vi "Get Slaves.vi"(8 "error in (no error)":errorcluster, 11 "EtherCAT Master in":T3 {"VS ref" format="%.0x"}) -> (0 "error out":errorcluster, 1 "ECAT Generic Slaves":T2(array[cluster]) {"VS ref" format="%.0x"}, 2 "ECAT Slaves":T2(array[cluster]) {"VS ref" format="%.0x"}, 3 "EtherCAT Master out":T3 {"VS ref" format="%.0x"}, 4 "ECAT REM Slaves":T2(array[cluster]) {"VS ref" format="%.0x"})   [LabVIEW 2019, in "SEECD Engine.lvlib"]
uses:
  SEECD Engine.lvlib
  <vilib>/NI VeriStand/Custom Device API/Custom Device Item Ref.ctl
  Shared/Globals/Scan Engine GUIDs.vi
  <vilib>/NI VeriStand/Custom Device API/Custom Device API.lvlib
  Shared/SEECD Shared.lvlib
  <resource>/objmgr/IndComECAT.rc
  <vilib>/NI VeriStand/Custom Device Tools/Custom Device Utility Library/Custom Device Utility Library.lvlib
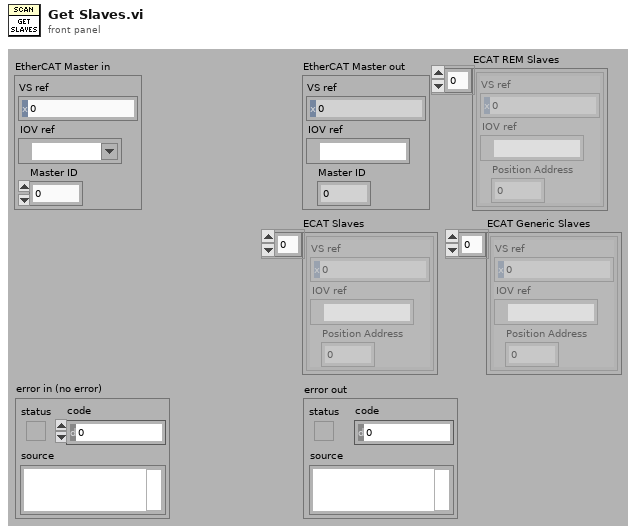
[diagram p1: front panel]
types:
  T1 = typedef "Custom Device API.lvlib/Custom Device Item Ref.ctl" = u64
  T2 = cluster{"VS ref":T1, "IOV ref":refnum<k21>, "Position Address":u16}[]
  T3 = cluster{"VS ref":T1, "IOV ref":refnum<k21>, "Master ID":u32}
  T4 = cluster{"ECAT Slave refs":T1[], "All ECAT Slaves":refnum<k21>[]}
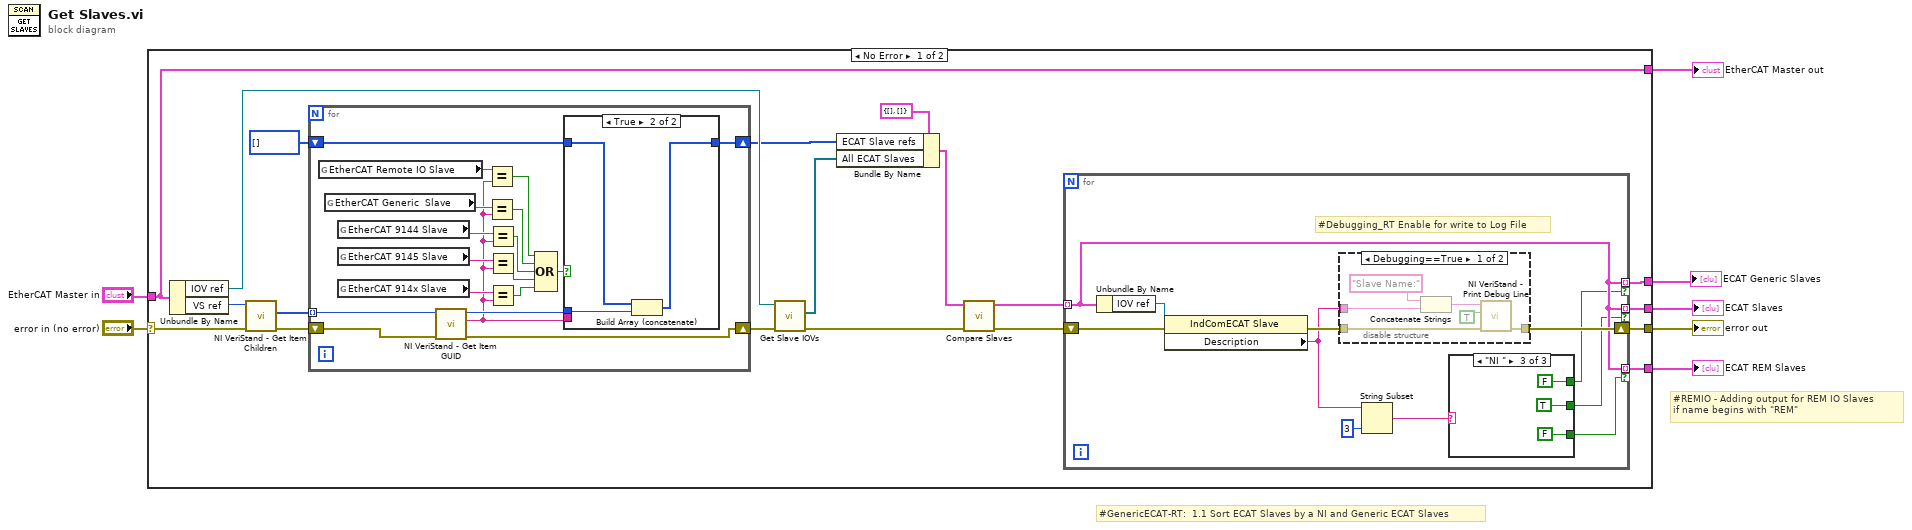
[diagram p0: block diagram]
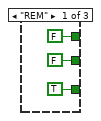
[diagram p3: hidden frame]
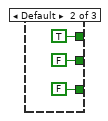
[diagram p4: hidden frame]
diagram:
  # "#REMIO - Adding output for REM IO Slaves\nif name begins with \"REM\""
  # "#GenericECAT-RT:  1.1 Sort ECAT Slaves by a NI and Generic ECAT Slaves"
  n1 = case shown="No Error" "error in (no error)" {
    selector: "error in (no error)" -> [w23 w77]
    tunnel: [w10 w77] -> w7
    tunnel: [w16 w76] -> w4
    tunnel: "EtherCAT Master in" -> [w16 w76]
    tunnel: [w12 _] -> w3
    tunnel: [w11 _] -> w2
    tunnel: [w8 _] -> w1
    frame No Error {
      n2 = Unbundle By Name(w16) -> ("IOV ref"=w18:refnum<k21>, "VS ref"=w19:T1)
      n3 = call <vilib>:"NI VeriStand - Get Item Children.vi"("error in (no error)"=w23, "Item Ref in"=w19) -> ("error out"=w24:errorcluster, "Child Refs"=w25:T1[])  [unwired: 6 in, 2 out]
      n4 = for {
        tunnel: w25 -> [w71] mode=indexing
        shift-right: [w67] -> w9
        shift-left: T1[] [] -> [w68]
        shift-right: [w65] -> w21
        shift-left: w24 -> [w66]
        n5 = global read "Scan Engine GUIDs.vi" "EtherCAT Remote IO Slave"() -> (w56:string)
        n6 = global read "Scan Engine GUIDs.vi" "EtherCAT Generic  Slave"() -> (w63:string)
        n7 = global read "Scan Engine GUIDs.vi" "EtherCAT 9144 Slave"() -> (w61:string)
        n8 = global read "Scan Engine GUIDs.vi" "EtherCAT 9145 Slave"() -> (w62:string)
        n9 = global read "Scan Engine GUIDs.vi" "EtherCAT 914x Slave"() -> (w70:string)
        n10 = call <vilib>:"NI VeriStand - Get Item GUID.vi"("error in (no error)"=w66, "Item Ref in"=w71) -> ("error out"=w65:errorcluster, "GUID"=w55:string, "Item Ref out"=w69:T1)  [unwired: 7 in]
        n11 = Equal?(x=w56, y=w55) -> (x = y?=w54:bool)
        n12 = Equal?(x=w63, y=w55) -> (x = y?=w57:bool)
        n13 = Equal?(x=w61, y=w55) -> (x = y?=w58:bool)
        n14 = Equal?(x=w62, y=w55) -> (x = y?=w59:bool)
        n15 = Equal?(x=w70, y=w55) -> (x = y?=w60:bool)
        n16 = Compound Arithmetic op=OR(w54, w57, w58, w59, w60) -> (w64:bool)
        n17 = case shown="True" w64 {
          tunnel: w69 -> [_ w74]
          tunnel: w68 -> [w72 w75]
          tunnel: [w72 w73] -> w67
          tunnel: w55 -> [_ _]
          frame False {
          }
          frame True {
            n18 = Build Array (concatenate)(w75, w74) -> (w73:T1[])
          }
        }
      }
      n19 = call "Get Slave IOVs.vi"("error in (no error)"=w21, "ECAT Master in"=w18) -> ("error IO"=w15:errorcluster, "All Slaves"=w20:refnum<k21>[])  [unwired: 7 in, 1 out]
      n20 = Bundle By Name(cluster=T4 {"ECAT Slave refs"=[], "All ECAT Slaves"=[]} ("ECAT Slaves"), "ECAT Slave refs"=w9, "All ECAT Slaves"=w20) -> (w17:T4)
      n21 = call "Compare Slaves.vi"("error in (no error)"=w15, "ECAT Slaves in"=w17) -> ("error out"=w13:errorcluster, "ECAT Slaves out"=w14:T2)  [unwired: 8 in]
      n22 = for {
        tunnel: w14 -> [w30] mode=indexing
        tunnel: [w30] -> w11 mode=indexing if=w29
        tunnel: [w30] -> w12 mode=indexing if=w28
        shift-right: [w35] -> w10
        shift-left: w13 -> [w36]
        tunnel: [w30] -> w8 mode=indexing if=w27
        # "#Debugging_RT Enable for write to Log File"
        n23 = Unbundle By Name(w30) -> ("IOV ref"=w37:refnum<k21>)
        n24 = property class="IndComECAT Slave"(reference=w37, error in=w36) -> (error out=w34:errorcluster, "Description"=w32:string)  [unwired: 1 out]
        n25 = disable-structure shown="Debugging==True" {
          disable-tunnel: [w41 w44] -> w35
          disable-tunnel: w34 -> [w39 w44]
          disable-tunnel: w32 -> [w38 _]
          frame condition #0 {
            n26 = Concatenate Strings("Slave Name:", w38) -> (w42:string)
            n27 = call <vilib>:"NI VeriStand - Print Debug Line.vi"("error in (no error)"=w39, "Add to log file? (F)"=TRUE ("Add to log file? (T)"), "Message"=w42) -> ("error out"=w41:errorcluster)  [unwired: 8 in]
          }
          frame condition #1 (active) {
          }
        }
        n28 = String Subset(string=w32, length (rest)=3 ("Länge (Rest)")) -> (substring=w31:string)  [unwired: 1 in]
        n29 = case shown="\"NI \"" w31 {
          tunnel: [FALSE TRUE FALSE] -> w29
          tunnel: [FALSE FALSE TRUE] -> w28
          tunnel: [TRUE FALSE FALSE] -> w27
          frame "REM" {
          }
          frame Default {
          }
          frame "NI " {
          }
        }
      }
    }
    frame Error {
    }
  }
  "error out" <- w7
  "EtherCAT Master out" <- w4
  "ECAT Slaves" <- w3
  "ECAT Generic Slaves" <- w2
  "ECAT REM Slaves" <- w1
